vi "half adder.vi"() -> ()   [LabVIEW 2025]
panel:
  in  "cin":bool
  out "carry":bool
  out "sum":bool
  in  "b":bool
  in  "a":bool
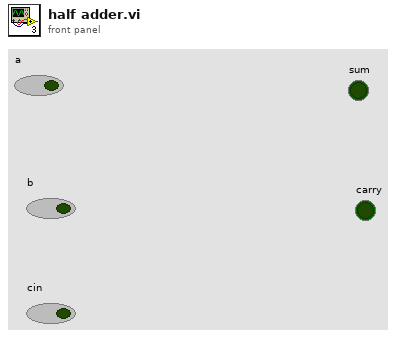
[diagram p1: front panel]
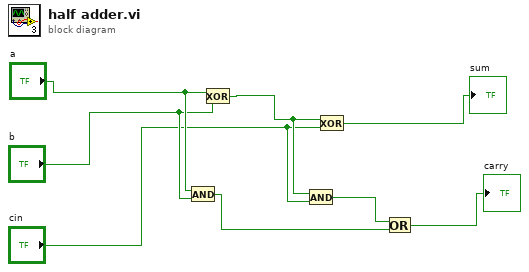
[diagram p0: block diagram]
diagram:
  n1 = And(x="a", y="b") -> (x .and. y?=w3:bool)
  n2 = Exclusive Or(1:"b", 2:"a") -> (0:w5:bool)
  n3 = And(x=w5, y="cin") -> (x .and. y?=w2:bool)
  n4 = Exclusive Or(1:"cin", 2:w5) -> (0:→"sum":bool)
  n5 = Or(x=w2, y=w3) -> (x .or. y?=→"carry":bool)
